vi "GetType.vi"(8 "error in (no error)":errorcluster, 11 "Fetch Msg":refnum<class "Fetch Msg.lvclass">) -> (0 "error out":errorcluster, 2 "Data Sample":variant, 3 "Fetch Msg":refnum<class "Fetch Msg.lvclass">)   [LabVIEW 2015, in "CS++DMM.lvlib" / "Fetch Msg.lvclass"]
uses:
  Fetch Msg.lvclass
  Fetch Msg.lvclass/Fetch Msg.ctl
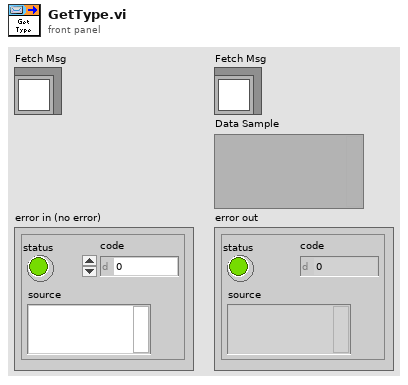
[diagram p1: front panel]
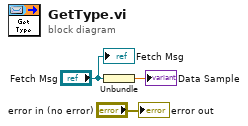
[diagram p0: block diagram]
diagram:
  n1 = Unbundle("Fetch Msg") -> (→"Data Sample":dbl[unit])
  "error out" <- "error in (no error)"
  "Fetch Msg" <- "Fetch Msg"
